vi "DFConfig Get First Tag.vi"(11 "String":string) -> (0 "End Tag":string, 1 "InnerString":string, 2 "Start Tag":string, 3 "After tag":string, 4 "No Tag?":bool)   [LabVIEW 2011]
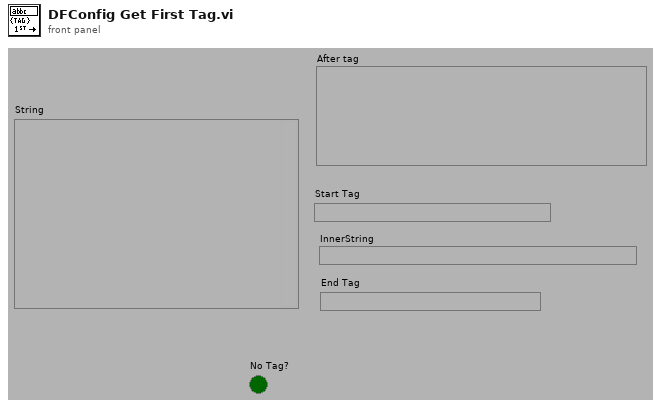
[diagram p1: front panel]
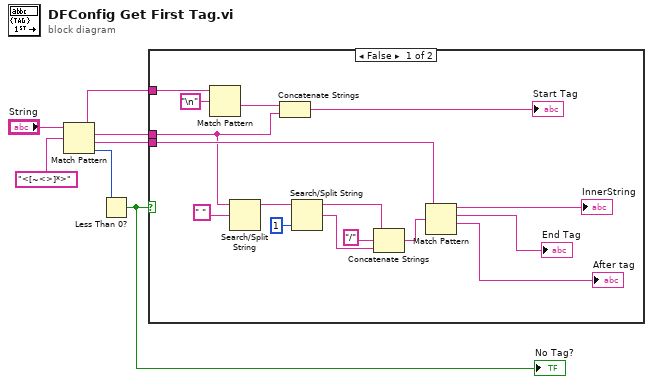
[diagram p0: block diagram]
diagram:
  n1 = Match Pattern(string="String", regular expression="<[~<>]*>") -> (before substring=w1:string, match substring=w4:string, after substring=w6:string, offset past match=w3:i32)  [unwired: 1 out]
  n2 = Less Than 0?(x=w3) -> (x < 0?=w2:bool)
  "No Tag?" <- w2
  n3 = case shown="False" w2 {
    tunnel: w6 -> [w23 _]
    tunnel: w4 -> [w10 _]
    tunnel: w1 -> [w12 _]
    frame False {
      n4 = Match Pattern(string=w12, regular expression="\n") -> (after substring=w11:string)  [unwired: 4 out]
      n5 = Search/Split String(string=w10, search string/char (-)=" ") -> (substring before match=w20:string)  [unwired: 3 out]
      n6 = Concatenate Strings(w11, w10) -> (→"Start Tag":string)
      n7 = Search/Split String(string=w20, offset (0)=1) -> (substring before match=w17:string, match + rest of string=w18:string)  [unwired: 2 out]
      n8 = Concatenate Strings(w17, "/", w18) -> (w16:string)
      n9 = Match Pattern(string=w23, regular expression=w16) -> (before substring=→"InnerString":string, match substring=→"End Tag":string, after substring=→"After tag":string)  [unwired: 2 out]
    }
    frame True {
    }
  }
